vi "Bundle AOL parameters at start.vi"(6 "Case name string":string, 8 "error in (no error)":errorcluster) -> (0 "error out":errorcluster, 2 "cancelled":bool)   [LabVIEW 2020]
uses:
  Typedefs/Imaging Protocols enum.ctl
  Typedefs/AOL modes.ctl
  Global Variables/gl_UI Ctrl Refs.vi
  Global Variables/General Globals.vi
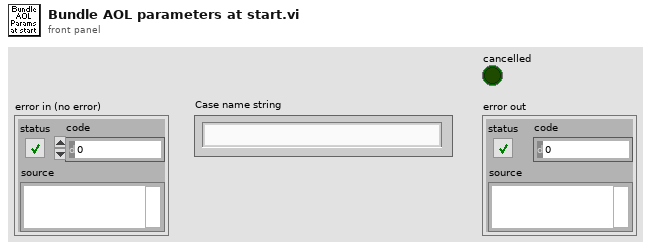
[diagram p1: front panel]
types:
  T1 = typedef "Imaging Protocols enum.ctl" = enum16{"AOL Z-Stack", "Motor Z Stack", "Parameter Sweep", "Functional Acquisition", "Single Plane Acquisition", "Volume Acquisition", "Live Imaging", "Live Plane Imaging", "Live Volume Imaging"}
  T2 = typedef "AOL modes.ctl" = enum16{"Raster", "Structural", "Pointing", "Mini Scan", "Alignment"}
  T3 = typedef "UI ctrl refs cluster.ctl" = cluster{"Top level VI path":path, "Top level VI ref":refnum<vi>, "User menu ref":refnum<k9>, "Sub Panel control":refnum<vi>, "Imaging Param Tab":refnum<vi>, "Occurrence-Start drivers":refnum<k4>, "Occurrence-Speed logging initialised":refnum<k4>, "Occurrence-XYZ stage initialised":refnum<k4>, "Exit button":refnum<vi>, "Status ind":refnum<vi>, "Set as origin":refnum<vi>, "Speed Logging":refnum<vi>, "Time Lapse":refnum<vi>, "Live Imaging":refnum<vi>, "AOL Z Stack":refnum<vi>, "Motor Z Stack":refnum<vi>, "Funct Acq button":refnum<vi>, "Hard Shutter":refnum<vi>, "Virtual Shutter":refnum<vi>, "Laser Power":refnum<vi>, "AOL Mode":refnum<vi>, "Frame Size":refnum<vi>, "Field of View":refnum<vi>, "Dwell Time":refnum<vi>, "Zoom":refnum<vi>, "AOL Z":refnum<vi>, "Objective":refnum<vi>, "Axis":refnum<vi>, "Paths & Names":refnum<vi>, "Experiment folder path (ind.)":refnum<vi>, "Last State (Ind.)":refnum<vi>, "Averages":refnum<vi>, "Angle (degrees)":refnum<vi>, "X centre":refnum<vi>, "Y centre":refnum<vi>, "Plane Mode":refnum<vi>, "# Planes":refnum<vi>, "Z Start":refnum<vi>, "Z Stop":refnum<vi>, "Z Step":refnum<vi>, "PMT 1":refnum<vi>, "PMT 2":refnum<vi>, "Stage XYZ Position":refnum<vi>, "Pockels@Z Start":refnum<vi>, "Pockels@Z Stop":refnum<vi>, "Obtain Z Start":refnum<vi>, "Obtain Z Stop":refnum<vi>, "Live stim.trig.period":refnum<vi>, "Live stim.trig.enable":refnum<vi>, "Movement Correction":refnum<vi>, "Load Reference Image":refnum<vi>, "XY Stage Move":refnum<vi>, "MovCor Cluster":refnum<vi>, "RefDAQParam":refnum<vi>, "Funct. Acq. Pockels Modulation":refnum<vi>, "Ref Laser Power":refnum<vi>, "Enable Video Recording":refnum<vi>, "Video Record-Live Imaging":refnum<vi>, "Video Record-Funct acq":refnum<vi>, "Reference Source":refnum<vi>, "AOL Z-stack Chirps Ready (ind)":refnum<vi>, "Target time between mov.cor. ref triggers (ms)":refnum<vi>, "Funct. Acq. Ref frame save":refnum<vi>, "Tracking button":refnum<vi>, "Show ref plots window":refnum<vi>, "Center freq ind (nm)":refnum<vi>, "Pickup mode (ind)":refnum<vi>, "Logging queue (ind)":refnum<vi>, "Back aperture power (ind.)":refnum<vi>, "Power after objective (ind.)":refnum<vi>, "Switch user":refnum<vi>, "Ls1 Conn. Status":refnum<vi>, "Ls1Tuning Status":refnum<vi>, "Ls1 Faults":refnum<vi>, "Ls1 Connection":refnum<vi>, "Ls1 Mode":refnum<vi>, "Ls1 POWER [mW]":refnum<vi>, "Ls1Shutter":refnum<vi>, "Ls1 Wavelength":refnum<vi>, "Ls1 Note":refnum<vi>, "Ls1 Confirm Wav":refnum<vi>, "Ls1 PreChrp Prism1":refnum<vi>, "Ls1 PreChrp Prism2":refnum<vi>, "Ls1 wav top Ind":refnum<vi>, "Ls1 power top Ind":refnum<vi>, "Ls1 Pump peak Hold":refnum<vi>, "Ls1 Status Ind":refnum<vi>, "Ls1 wav cancel":refnum<vi>, "Experiment Type":refnum<vi>, "Biology Information":refnum<vi>, "Camera recording status":refnum<vi>, "Optimise Obj. Pos.":refnum<vi>}
  T4 = typedef "AOL_Globals.ctl" = cluster{"Imaging Protocol":T1, "Number of POI":u16, "Number of Miniscans":u16, "Number of Trials":u16, "Number of Cycles ":u64, "# Averaged Frames":u16, "Laser power (%)":u8, "Pockels (V)":dbl, "Acquisition Length (sec)":dbl, "Fill time (us)":dbl, "POI Dwell time (us)":dbl, "Miniscan Dwell time per pixel (us)":dbl, "PMT 1":dbl, "PMT 2":dbl, "Back Apperture (mA)":dbl, "Frame Size":T5, "Center Frequency":dbl, "Field of View (um)":dbl, "Field of View (norm)":dbl, "DwellTime (us)":dbl, "Ref Dwell Time (us)":dbl, "Wavelength (nm)":dbl, "Zoom":dbl, "AOL Z":dbl, "AOL Mode":T2, "GridXY":dbl, "GridZ":dbl, "TriggerPeriod (sec)":dbl, "Number of Pixels in Miniscan":u16, "Experiment folder path":path, "X centre":dbl, "Y centre":dbl, "Angle (degrees)":dbl, "Angle Xs (degrees)":dbl, "Angle Ys (degrees)":dbl, "Plane Mode":T6, "Threshold":u16[], "Regenerate Chirps":bool, "Rectangle ROI length (pixels)":u16, "Rectangle ROI height (pixels)":u16, "AOD fill":u16, "StartupDelay":i32, "Samples Wait after Trigger":u16, "Slip Cycle":u32, "Add Cycle":bool, "Functional Mode":T7, "Z Start":dbl, "Z Stop":dbl, "# Planes":i32, "Total Pixels":i32, "Variable Miniscan Pixels":u16[], "Use Variable Length":bool, "Use Variable Resolution":bool, "Laser power (%) at Z Start":u8, "Laser power (%) at Z Stop":u8, "Ref Z Step":i8}
  T5 = typedef "Frame Size.ctl" = u16
  T6 = typedef "Plane Mode.ctl" = u16
  T7 = typedef "Functional Mode.ctl" = enum16{"Point", "Line", "Patch", "Plane", "Volume"}
  T8 = typedef "Laser control knob.ctl" = u16
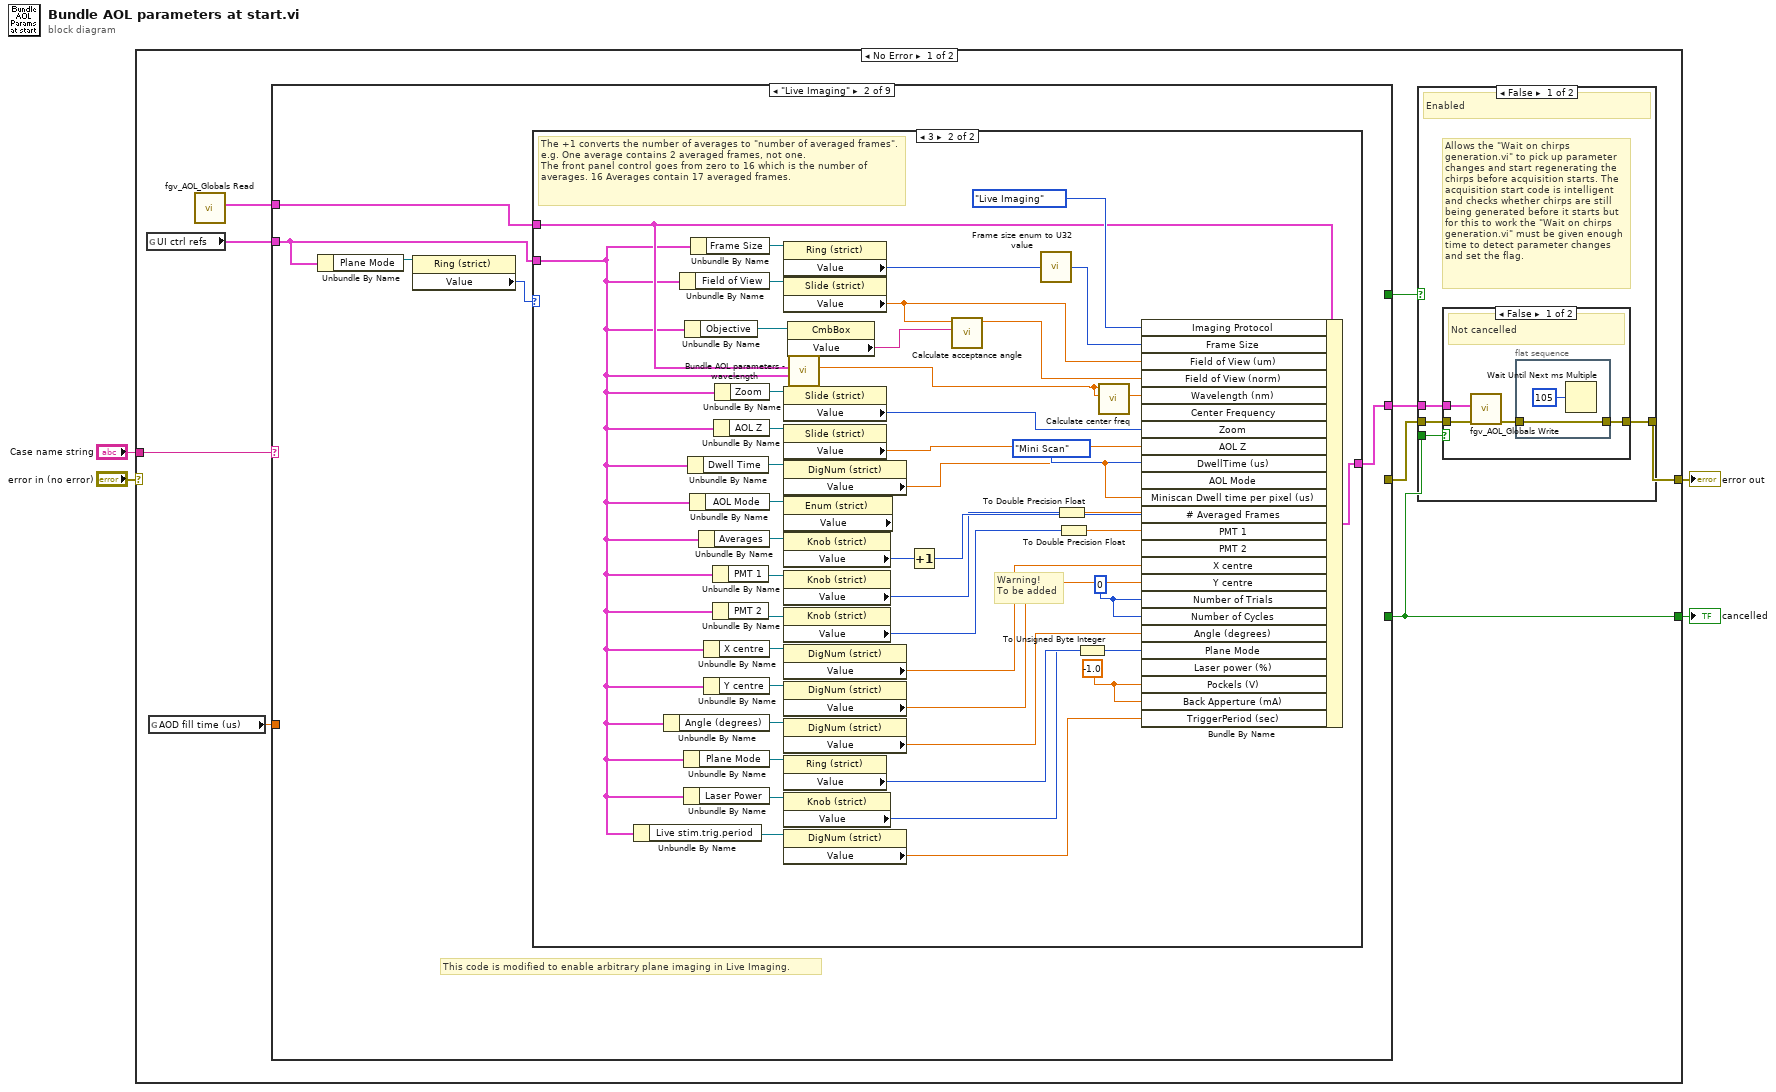
[diagram p0: block diagram]
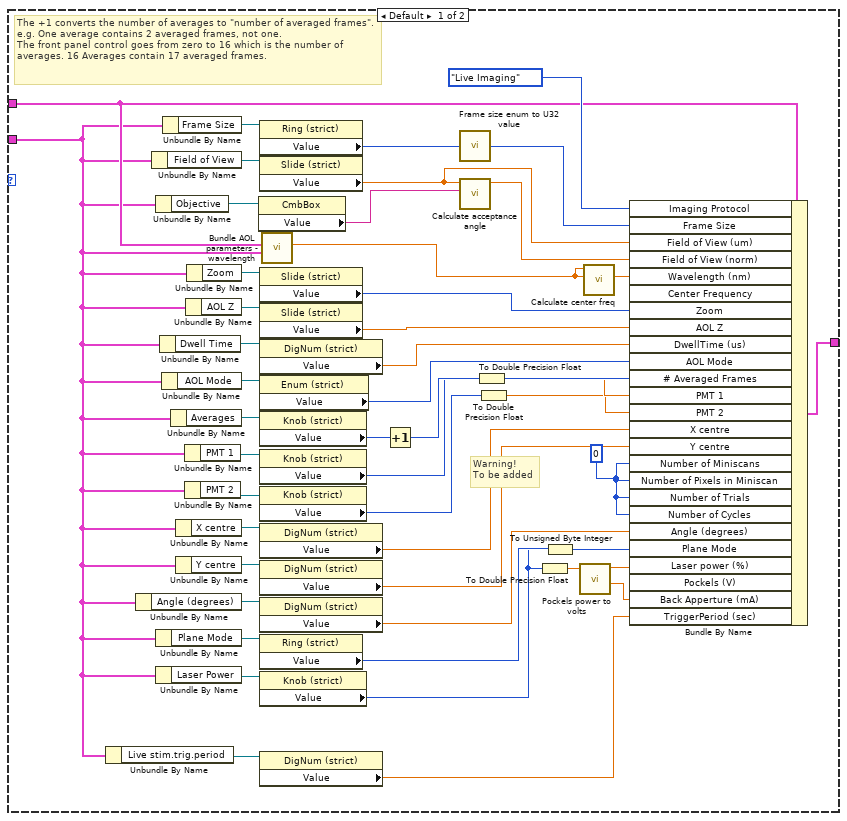
[diagram p5: hidden frame]
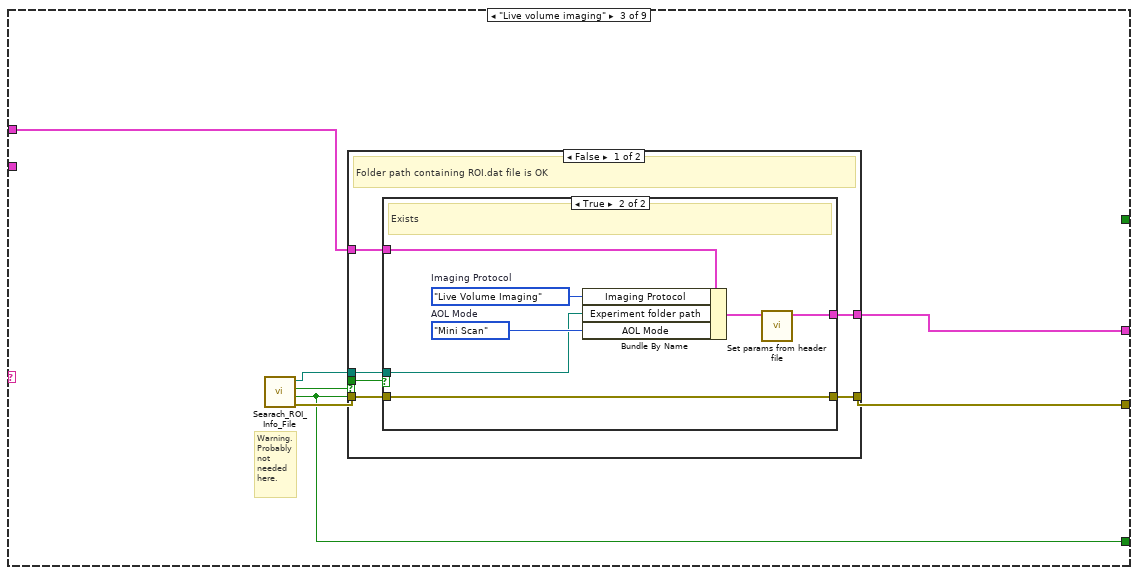
[diagram p6: hidden frame]
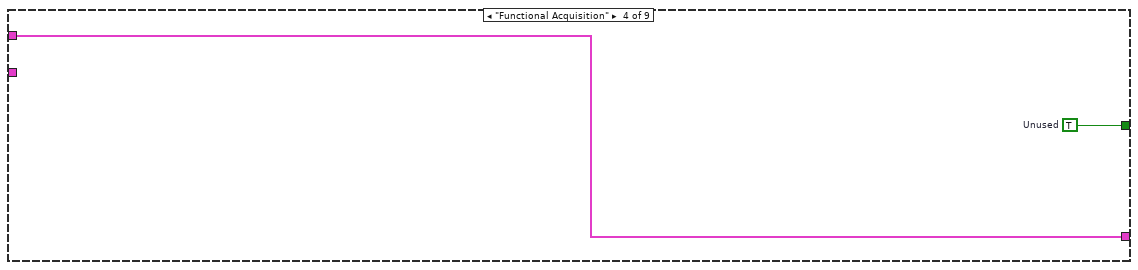
[diagram p9: hidden frame]
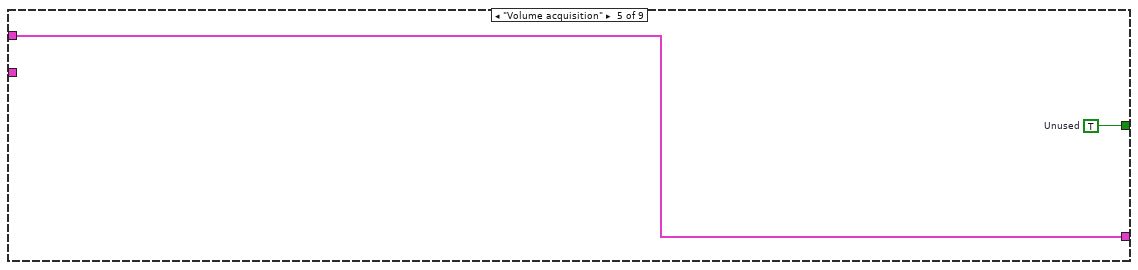
[diagram p10: hidden frame]
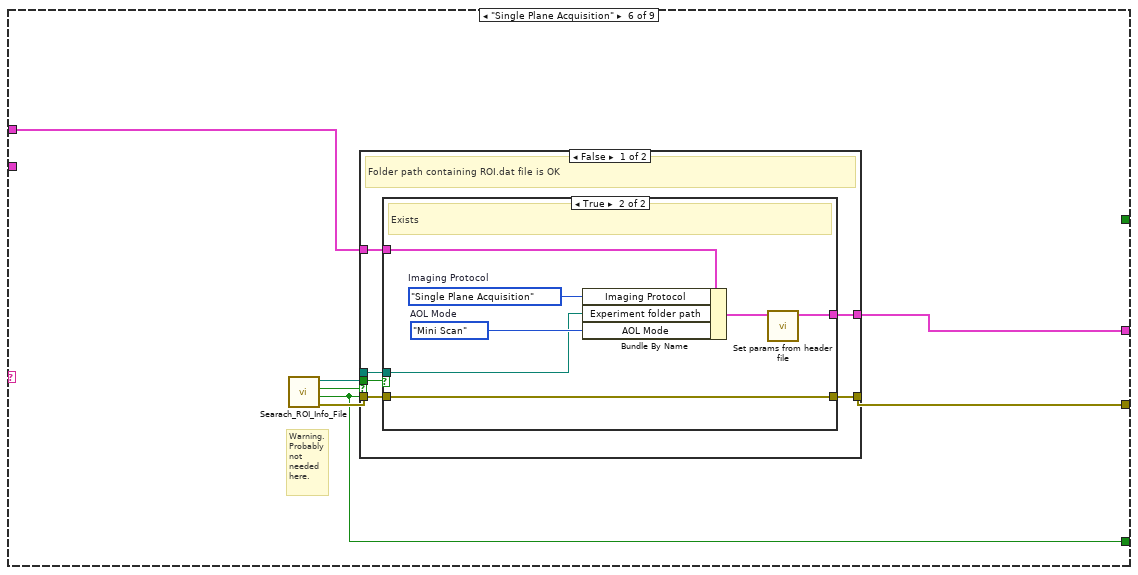
[diagram p11: hidden frame]
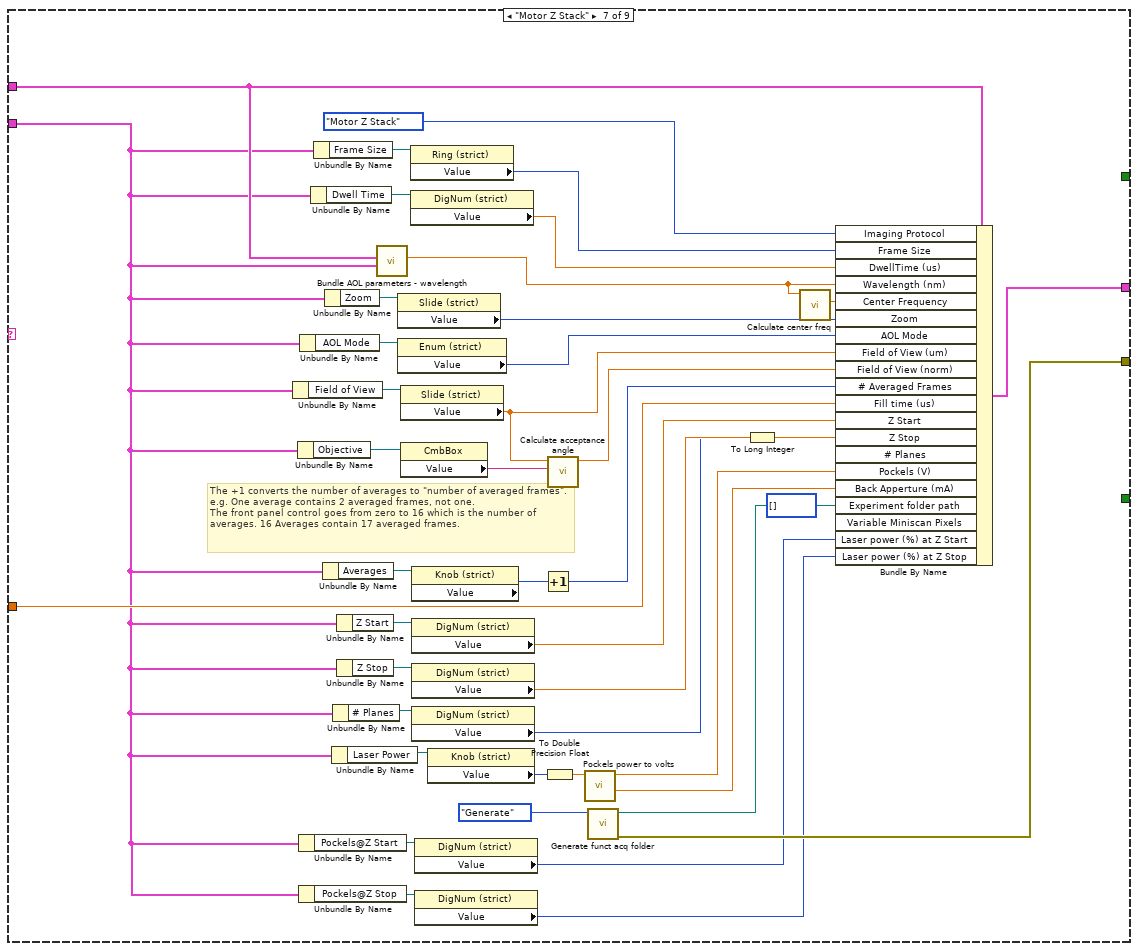
[diagram p14: hidden frame]
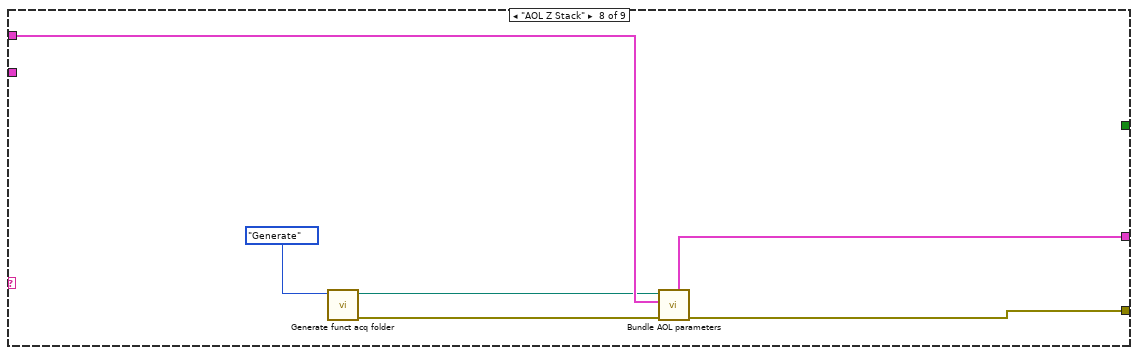
[diagram p15: hidden frame]
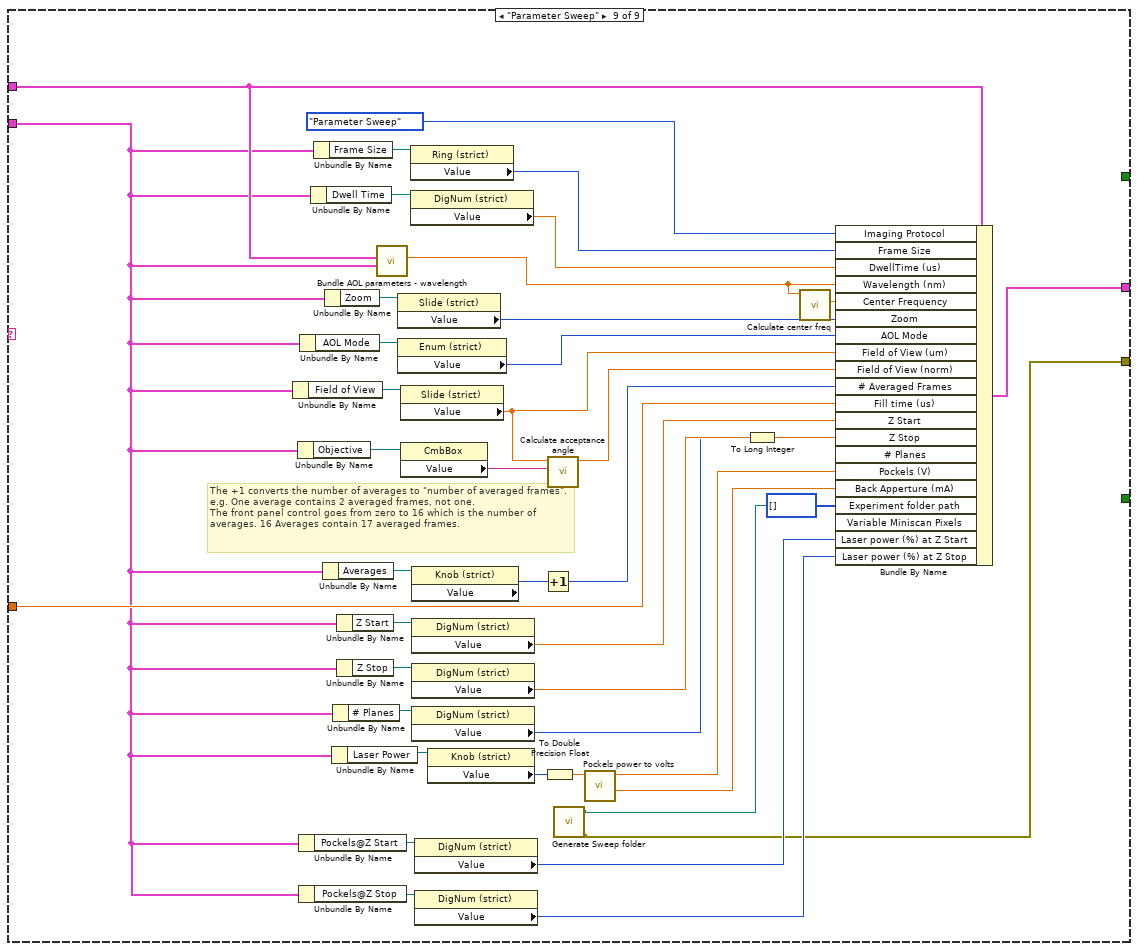
[diagram p16: hidden frame]
diagram:
  n1 = case shown="No Error" "error in (no error)" {
    selector: "error in (no error)" -> [_ w267]
    tunnel: [w13 w267] -> w1
    tunnel: "Case name string" -> [w10 _]
    tunnel: [w6 _] -> w2
    frame No Error {
      n2 = global read "gl_UI Ctrl Refs.vi" "UI ctrl refs"() -> (w9:T3)
      n3 = global read "General Globals.vi" "AOD fill time (us)"() -> (w8:dbl)
      n4 = call "fgv_AOL_Globals Read.vi"() -> ("AOL_Globals"=w11:T4)  [unwired: 9 in, 2 out]
      n5 = case shown="\"Live Imaging\"" w10 {
        tunnel: [w25 w29 w127 w149 w152 w155 w203 w222 w251] -> w12
        tunnel: w11 -> [w25 w30 w128 w149 w152 w156 w194 w223 w243]
        tunnel: w9 -> [_ w28 _ _ _ _ w180 _ w230]
        tunnel: w8 -> [_ _ _ _ _ _ w200 _ w249]
        tunnel: [_ _ w126 _ _ w154 w202 w221 w227] -> w7
        tunnel: [_ _ w125 _ _ w153 _ _ _] -> w6
        tunnel: [_ _ _ w150 w151 _ _ _ _] -> w5
        frame Default {
        }
        frame "Live Imaging" {
          # "This code is modified to enable arbitrary plane imaging in Live Imaging."
          n6 = Unbundle By Name(w28) -> ("Plane Mode"=w27:refnum<vi>)
          n7 = property on="Property Node" class="Ring (strict)"(reference=w27) -> ("Value"=w26:T6)  [unwired: 1 in, 2 out]
          n8 = case shown="3" w26 {
            tunnel: w30 -> [w41 w83]
            tunnel: [w57 w104] -> w29
            tunnel: w28 -> [w37 w79]
            frame Default {
              w78 = u16 0 ("Number of Miniscans")
              # "Warning!\nTo be added"
              # "The +1 converts the number of averages to \"number of averaged frames\". e.g. One average contains 2 averaged frames, not one.\nThe front panel control goes from zero to 16 which is the number of averages. 16 Averages contain 17 averaged frames."
              n9 = Unbundle By Name(w37) -> ("Live stim.trig.period"=w45:refnum<vi>)
              n10 = Unbundle By Name(w37) -> ("Angle (degrees)"=w61:refnum<vi>)
              n11 = Unbundle By Name(w37) -> ("Field of View"=w67:refnum<vi>)
              n12 = Unbundle By Name(w37) -> ("Objective"=w39:refnum<vi>)
              n13 = Unbundle By Name(w37) -> ("Plane Mode"=w58:refnum<vi>)
              n14 = Unbundle By Name(w37) -> ("Laser Power"=w53:refnum<vi>)
              n15 = Unbundle By Name(w37) -> ("Dwell Time"=w64:refnum<vi>)
              n16 = Unbundle By Name(w37) -> ("AOL Mode"=w63:refnum<vi>)
              n17 = Unbundle By Name(w37) -> ("Frame Size"=w68:refnum<vi>)
              n18 = Unbundle By Name(w37) -> ("Averages"=w62:refnum<vi>)
              n19 = Unbundle By Name(w37) -> ("X centre"=w60:refnum<vi>)
              n20 = Unbundle By Name(w37) -> ("Y centre"=w59:refnum<vi>)
              n21 = Unbundle By Name(w37) -> ("PMT 1"=w51:refnum<vi>)
              n22 = Unbundle By Name(w37) -> ("PMT 2"=w50:refnum<vi>)
              n23 = Unbundle By Name(w37) -> ("AOL Z"=w65:refnum<vi>)
              n24 = Unbundle By Name(w37) -> ("Zoom"=w66:refnum<vi>)
              n25 = property on="Property Node" class="CmbBox"(reference=w39) -> ("Value"=w38:string)  [unwired: 1 in, 2 out]
              n26 = property on="Property Node" class="Ring (strict)"(reference=w68) -> ("Value"=w55:T5)  [unwired: 1 in, 2 out]
              n27 = property on="Property Node" class="Slide (strict)"(reference=w67) -> ("Value"=w31:sgl)  [unwired: 1 in, 2 out]
              n28 = property on="Property Node" class="Slide (strict)"(reference=w66) -> ("Value"=w73:i8)  [unwired: 1 in, 2 out]
              n29 = property on="Property Node" class="Slide (strict)"(reference=w65) -> ("Value"=w70:sgl)  [unwired: 1 in, 2 out]
              n30 = property on="Property Node" class="DigNum (strict)"(reference=w64) -> ("Value"=w71:dbl)  [unwired: 1 in, 2 out]
              n31 = property on="Property Node" class="Enum (strict)"(reference=w63) -> ("Value"=w77:T2)  [unwired: 1 in, 2 out]
              n32 = property on="Property Node" class="Knob (strict)"(reference=w62) -> ("Value"=w72:u16)  [unwired: 1 in, 2 out]
              n33 = property on="Property Node" class="Knob (strict)"(reference=w51) -> ("Value"=w49:T8)  [unwired: 1 in, 2 out]
              n34 = property on="Property Node" class="Knob (strict)"(reference=w50) -> ("Value"=w48:T8)  [unwired: 1 in, 2 out]
              n35 = property on="Property Node" class="DigNum (strict)"(reference=w60) -> ("Value"=w74:dbl)  [unwired: 1 in, 2 out]
              n36 = property on="Property Node" class="DigNum (strict)"(reference=w59) -> ("Value"=w75:dbl)  [unwired: 1 in, 2 out]
              n37 = property on="Property Node" class="DigNum (strict)"(reference=w61) -> ("Value"=w69:dbl)  [unwired: 1 in, 2 out]
              n38 = property on="Property Node" class="Ring (strict)"(reference=w58) -> ("Value"=w43:T6)  [unwired: 1 in, 2 out]
              n39 = property on="Property Node" class="Knob (strict)"(reference=w53) -> ("Value"=w33:T8)  [unwired: 1 in, 2 out]
              n40 = property on="Property Node" class="DigNum (strict)"(reference=w45) -> ("Value"=w44:dbl)  [unwired: 1 in, 2 out]
              n41 = call "Bundle AOL parameters - wavelength.vi"("UI ctrl refs"=w37, "AOL_Globals in"=w41) -> ("Wavelength"=w40:dbl)  [unwired: 9 in]
              n42 = Increment(x=w72) -> (x+1=w56:u16)
              n43 = call "Frame size enum to U32 value.vi"("Value"=w55) -> ("Frame Size U32"=w54:u32)
              n44 = call "Calculate acceptance angle.vi"("Objective"=w38, "FOV (true)"=w31) -> ("Acceptance Angle (mrad)"=w36:dbl)  [unwired: 8 in, 1 out]
              n45 = To Double Precision Float(number=w49) -> (double precision float=w47:dbl)
              n46 = To Double Precision Float(number=w48) -> (double precision float=w46:dbl)
              n47 = To Double Precision Float(number=w33) -> (double precision float=w32:dbl)
              n48 = To Unsigned Byte Integer(number=w33) -> (unsigned 8bit integer=w52:u8)
              n49 = call "Pockels power to volts.vi"("Pockels power (%)"=w32) -> ("Back-aperture power (mW)"=w34:dbl, "Pockels control voltage (V)"=w35:dbl)  [unwired: 8 in, 1 out]
              n50 = call "Calculate center freq.vi"("UI Wavelength"=w40) -> ("Centre frequency (MHz)"=w42:dbl)  [unwired: 9 in, 1 out]
              n51 = Bundle By Name(cluster=w41, "Imaging Protocol"=Imaging_Protocols_enum."Live Imaging" ("Imaging Mode"), "Frame Size"=w54, "Field of View (um)"=w31, "Field of View (norm)"=w36, "Wavelength (nm)"=w40, "Center Frequency"=w42, "Zoom"=w73, "AOL Z"=w70, "DwellTime (us)"=w71, "AOL Mode"=w77, "# Averaged Frames"=w56, "PMT 1"=w47, "PMT 2"=w46, "X centre"=w74, "Y centre"=w75, "Number of Miniscans"=w78, "Number of Pixels in Miniscan"=w78, "Number of Trials"=w78, "Number of Cycles"=w78, "Angle (degrees)"=w69, "Plane Mode"=w43, "Laser power (%)"=w52, "Pockels (V)"=w35, "Back Apperture (mA)"=w34, "TriggerPeriod (sec)"=w44) -> (w57:T4)
            }
            frame 3 {
              w91 = -1.0 ("Pockels")
              w124 = u16 0 ("Number of Miniscans")
              # "Warning!\nTo be added"
              # "The +1 converts the number of averages to \"number of averaged frames\". e.g. One average contains 2 averaged frames, not one.\nThe front panel control goes from zero to 16 which is the number of averages. 16 Averages contain 17 averaged frames."
              n52 = Unbundle By Name(w79) -> ("Live stim.trig.period"=w89:refnum<vi>)
              n53 = Unbundle By Name(w79) -> ("Angle (degrees)"=w108:refnum<vi>)
              n54 = Unbundle By Name(w79) -> ("Field of View"=w114:refnum<vi>)
              n55 = Unbundle By Name(w79) -> ("Plane Mode"=w105:refnum<vi>)
              n56 = Unbundle By Name(w79) -> ("Laser Power"=w100:refnum<vi>)
              n57 = Unbundle By Name(w79) -> ("Objective"=w84:refnum<vi>)
              n58 = Unbundle By Name(w79) -> ("Dwell Time"=w111:refnum<vi>)
              n59 = Unbundle By Name(w79) -> ("AOL Mode"=w110:refnum<vi>)
              n60 = Unbundle By Name(w79) -> ("Frame Size"=w115:refnum<vi>)
              n61 = Unbundle By Name(w79) -> ("Averages"=w109:refnum<vi>)
              n62 = Unbundle By Name(w79) -> ("X centre"=w107:refnum<vi>)
              n63 = Unbundle By Name(w79) -> ("Y centre"=w106:refnum<vi>)
              n64 = Unbundle By Name(w79) -> ("PMT 1"=w97:refnum<vi>)
              n65 = Unbundle By Name(w79) -> ("PMT 2"=w96:refnum<vi>)
              n66 = Unbundle By Name(w79) -> ("AOL Z"=w112:refnum<vi>)
              n67 = Unbundle By Name(w79) -> ("Zoom"=w113:refnum<vi>)
              n68 = property on="Property Node" class="Ring (strict)"(reference=w115) -> ("Value"=w102:T5)  [unwired: 1 in, 2 out]
              n69 = property on="Property Node" class="Slide (strict)"(reference=w114) -> ("Value"=w82:sgl)  [unwired: 1 in, 2 out]
              n70 = property on="Property Node" class="Slide (strict)"(reference=w113) -> ("Value"=w120:i8)  [unwired: 1 in, 2 out]
              n71 = property on="Property Node" class="Slide (strict)"(reference=w112) -> ("Value"=w118:sgl)  [unwired: 1 in, 2 out]
              n72 = property on="Property Node" class="DigNum (strict)"(reference=w111) -> ("Value"=w87:dbl)  [unwired: 1 in, 2 out]
              n73 = property on="Property Node" class="Enum (strict)" props=["Value"](reference=w110) -> ()  [unwired: 1 in, 3 out]
              n74 = property on="Property Node" class="Knob (strict)"(reference=w109) -> ("Value"=w119:u16)  [unwired: 1 in, 2 out]
              n75 = property on="Property Node" class="Knob (strict)"(reference=w97) -> ("Value"=w95:T8)  [unwired: 1 in, 2 out]
              n76 = property on="Property Node" class="Knob (strict)"(reference=w96) -> ("Value"=w94:T8)  [unwired: 1 in, 2 out]
              n77 = property on="Property Node" class="DigNum (strict)"(reference=w107) -> ("Value"=w121:dbl)  [unwired: 1 in, 2 out]
              n78 = property on="Property Node" class="DigNum (strict)"(reference=w106) -> ("Value"=w122:dbl)  [unwired: 1 in, 2 out]
              n79 = property on="Property Node" class="DigNum (strict)"(reference=w108) -> ("Value"=w117:dbl)  [unwired: 1 in, 2 out]
              n80 = property on="Property Node" class="Ring (strict)"(reference=w105) -> ("Value"=w116:T6)  [unwired: 1 in, 2 out]
              n81 = property on="Property Node" class="Knob (strict)"(reference=w100) -> ("Value"=w99:T8)  [unwired: 1 in, 2 out]
              n82 = property on="Property Node" class="DigNum (strict)"(reference=w89) -> ("Value"=w88:dbl)  [unwired: 1 in, 2 out]
              n83 = property on="Property Node" class="CmbBox"(reference=w84) -> ("Value"=w81:string)  [unwired: 1 in, 2 out]
              n84 = call "Bundle AOL parameters - wavelength.vi"("UI ctrl refs"=w79, "AOL_Globals in"=w83) -> ("Wavelength"=w85:dbl)  [unwired: 9 in]
              n85 = Increment(x=w119) -> (x+1=w103:u16)
              n86 = call "Calculate acceptance angle.vi"("Objective"=w81, "FOV (true)"=w82) -> ("Acceptance Angle (mrad)"=w80:dbl)  [unwired: 8 in, 1 out]
              n87 = call "Frame size enum to U32 value.vi"("Value"=w102) -> ("Frame Size U32"=w101:u32)
              n88 = To Double Precision Float(number=w95) -> (double precision float=w93:dbl)
              n89 = To Double Precision Float(number=w94) -> (double precision float=w92:dbl)
              n90 = To Unsigned Byte Integer(number=w99) -> (unsigned 8bit integer=w98:u8)
              n91 = call "Calculate center freq.vi"("UI Wavelength"=w85) -> ("Centre frequency (MHz)"=w86:dbl)  [unwired: 9 in, 1 out]
              n92 = Bundle By Name(cluster=w83, "Imaging Protocol"=Imaging_Protocols_enum."Live Imaging" ("Imaging Mode"), "Frame Size"=w101, "Field of View (um)"=w82, "Field of View (norm)"=w80, "Wavelength (nm)"=w85, "Center Frequency"=w86, "Zoom"=w120, "AOL Z"=w118, "DwellTime (us)"=w87, "AOL Mode"=AOL_modes."Mini Scan", "Miniscan Dwell time per pixel (us)"=w87, "# Averaged Frames"=w103, "PMT 1"=w93, "PMT 2"=w92, "X centre"=w121, "Y centre"=w122, "Number of Trials"=w124, "Number of Cycles"=w124, "Angle (degrees)"=w117, "Plane Mode"=w116, "Laser power (%)"=w98, "Pockels (V)"=w91, "Back Apperture (mA)"=w91, "TriggerPeriod (sec)"=w88) -> (w104:T4)
            }
          }
        }
        frame "Live volume imaging" {
          # "Warning.\nProbably not needed here."
          n93 = call "Searach_ROI_Info_File.vi"() -> ("error out"=w130:errorcluster, "cancelled"=w125:bool, "exists"=w129:bool, "Experiment folder"=w131:path)  [unwired: 8 in]
          n94 = case shown="False" w125 {
            tunnel: w131 -> [w137 _]
            tunnel: w130 -> [w136 w147]
            tunnel: w129 -> [w135 _]
            tunnel: w128 -> [w134 w148]
            tunnel: [w133 w148] -> w127
            tunnel: [w132 w147] -> w126
            frame False {
              # "Folder path containing ROI.dat file is OK"
              n95 = case shown="True" w135 {
                tunnel: w137 -> [_ w144]
                tunnel: w136 -> [w139 w141]
                tunnel: w134 -> [w138 w143]
                tunnel: [w138 w140] -> w133
                tunnel: [w139 w141] -> w132
                frame False {
                  # "Deos not exist"
                }
                frame True {
                  w145 = AOL_modes."Mini Scan"  # AOL Mode
                  w146 = Imaging_Protocols_enum."Live Volume Imaging"  # Imaging Protocol
                  # "Exists"
                  n96 = Bundle By Name(cluster=w143, "Imaging Protocol"=w146, "Experiment folder path"=w144, "AOL Mode"=w145) -> (w142:T4)
                  n97 = call "Set params from header file.vi"("AOL_Globals in"=w142) -> ("AOL_Globals out"=w140:T4)  [unwired: 10 in]
                }
              }
            }
            frame True {
              # "Cancelled"
            }
          }
        }
        frame "Functional Acquisition" {
          w150 = TRUE  # Unused
        }
        frame "Volume acquisition" {
          w151 = TRUE  # Unused
        }
        frame "Single Plane Acquisition" {
          # "Warning.\nProbably not needed here."
          n98 = call "Searach_ROI_Info_File.vi"() -> ("error out"=w158:errorcluster, "cancelled"=w153:bool, "exists"=w157:bool, "Experiment folder"=w159:path)  [unwired: 8 in]
          n99 = case shown="False" w153 {
            tunnel: w159 -> [w165 _]
            tunnel: w158 -> [w164 w175]
            tunnel: w157 -> [w163 _]
            tunnel: w156 -> [w162 w176]
            tunnel: [w161 w176] -> w155
            tunnel: [w160 w175] -> w154
            frame False {
              # "Folder path containing ROI.dat file is OK"
              n100 = case shown="True" w163 {
                tunnel: w165 -> [_ w172]
                tunnel: w164 -> [w167 w170]
                tunnel: w162 -> [w166 w171]
                tunnel: [w166 w168] -> w161
                tunnel: [w167 w170] -> w160
                frame False {
                  # "Deos not exist"
                }
                frame True {
                  w173 = AOL_modes."Mini Scan"  # AOL Mode
                  w174 = Imaging_Protocols_enum."Single Plane Acquisition"  # Imaging Protocol
                  # "Exists"
                  n101 = Bundle By Name(cluster=w171, "Imaging Protocol"=w174, "Experiment folder path"=w172, "AOL Mode"=w173) -> (w169:T4)
                  n102 = call "Set params from header file.vi"("AOL_Globals in"=w169) -> ("AOL_Globals out"=w168:T4)  [unwired: 10 in]
                }
              }
            }
            frame True {
              # "Cancelled"
            }
          }
        }
        frame "Motor Z Stack" {
          # "The +1 converts the number of averages to \"number of averaged frames\". e.g. One average contains 2 averaged frames, not one.\nThe front panel control goes from zero to 16 which is the number of averages. 16 Averages contain 17 averaged frames."
          n103 = Unbundle By Name(w180) -> ("Field of View"=w212:refnum<vi>)
          n104 = Unbundle By Name(w180) -> ("Objective"=w192:refnum<vi>)
          n105 = Unbundle By Name(w180) -> ("Pockels@Z Start"=w182:refnum<vi>)
          n106 = Unbundle By Name(w180) -> ("Pockels@Z Stop"=w181:refnum<vi>)
          n107 = Unbundle By Name(w180) -> ("AOL Mode"=w213:refnum<vi>)
          n108 = Unbundle By Name(w180) -> ("Dwell Time"=w215:refnum<vi>)
          n109 = Unbundle By Name(w180) -> ("Frame Size"=w217:refnum<vi>)
          n110 = Unbundle By Name(w180) -> ("Averages"=w211:refnum<vi>)
          n111 = Unbundle By Name(w180) -> ("Zoom"=w214:refnum<vi>)
          n112 = Unbundle By Name(w180) -> ("Laser Power"=w188:refnum<vi>)
          n113 = Unbundle By Name(w180) -> ("# Planes"=w207:refnum<vi>)
          n114 = Unbundle By Name(w180) -> ("Z Start"=w205:refnum<vi>)
          n115 = Unbundle By Name(w180) -> ("Z Stop"=w206:refnum<vi>)
          n116 = call "Bundle AOL parameters - wavelength.vi"("UI ctrl refs"=w180, "AOL_Globals in"=w194) -> ("Wavelength"=w193:dbl)  [unwired: 9 in]
          n117 = property class="Slide (strict)"(reference=w214) -> ("Value"=w204:i8)  [unwired: 1 in, 2 out]
          n118 = property class="Enum (strict)"(reference=w213) -> ("Value"=w209:T2)  [unwired: 1 in, 2 out]
          n119 = property class="Slide (strict)"(reference=w212) -> ("Value"=w177:sgl)  [unwired: 1 in, 2 out]
          n120 = property on="Property Node" class="CmbBox"(reference=w192) -> ("Value"=w191:string)  [unwired: 1 in, 2 out]
          n121 = property class="Ring (strict)"(reference=w217) -> ("Value"=w216:u16)  [unwired: 1 in, 2 out]
          n122 = property class="DigNum (strict)"(reference=w215) -> ("Value"=w210:dbl)  [unwired: 1 in, 2 out]
          n123 = property class="Knob (strict)"(reference=w211) -> ("Value"=w208:u16)  [unwired: 1 in, 2 out]
          n124 = property class="DigNum (strict)"(reference=w205) -> ("Value"=w198:dbl)  [unwired: 1 in, 2 out]
          n125 = property class="DigNum (strict)"(reference=w206) -> ("Value"=w197:dbl)  [unwired: 1 in, 2 out]
          n126 = property class="DigNum (strict)"(reference=w207) -> ("Value"=w195:u16)  [unwired: 1 in, 2 out]
          n127 = property on="Property Node" class="DigNum (strict)"(reference=w182) -> ("Value"=w179:u16)  [unwired: 1 in, 2 out]
          n128 = property on="Property Node" class="DigNum (strict)"(reference=w181) -> ("Value"=w178:u16)  [unwired: 1 in, 2 out]
          n129 = property class="Knob (strict)"(reference=w188) -> ("Value"=w186:T8)  [unwired: 1 in, 2 out]
          n130 = Increment(x=w208) -> (x+1=w201:u16)
          n131 = To Double Precision Float(number=w186) -> (double precision float=w187:dbl)
          n132 = call "Calculate acceptance angle.vi"("Objective"=w191, "FOV (true)"=w177) -> ("Acceptance Angle (mrad)"=w190:dbl)  [unwired: 8 in, 1 out]
          n133 = call "Pockels power to volts.vi"("Pockels power (%)"=w187) -> ("Back-aperture power (mW)"=w184:dbl, "Pockels control voltage (V)"=w185:dbl)  [unwired: 8 in, 1 out]
          n134 = call "Generate funct acq folder.vi"("Function"=enum16{"Generate", "Obtain"}."Generate") -> ("error out"=w202:errorcluster, "Funct acq experiment folder path"=w189:path)  [unwired: 9 in]
          n135 = To Long Integer(number=w195) -> (32bit integer=w196:i32)
          n136 = call "Calculate center freq.vi"("UI Wavelength"=w193) -> ("Centre frequency (MHz)"=w199:dbl)  [unwired: 9 in, 1 out]
          n137 = Bundle By Name(cluster=w194, "Imaging Protocol"=Imaging_Protocols_enum."Motor Z Stack" ("Imaging Mode"), "Frame Size"=w216, "DwellTime (us)"=w210, "Wavelength (nm)"=w193, "Center Frequency"=w199, "Zoom"=w204, "AOL Mode"=w209, "Field of View (um)"=w177, "Field of View (norm)"=w190, "# Averaged Frames"=w201, "Fill time (us)"=w200, "Z Start"=w198, "Z Stop"=w197, "# Planes"=w196, "Pockels (V)"=w185, "Back Apperture (mA)"=w184, "Experiment folder path"=w189, "Variable Miniscan Pixels"=u16[] [], "Laser power (%) at Z Start"=w179, "Laser power (%) at Z Stop"=w178) -> (w203:T4)
        }
        frame "AOL Z Stack" {
          n138 = call "Generate funct acq folder.vi"("Function"=enum16{"Generate", "Obtain"}."Generate") -> ("error out"=w221:errorcluster, "Funct acq experiment folder path"=w220:path)  [unwired: 9 in]
          n139 = call "Bundle AOL parameters.vi"("AOL_Globals in"=w223, "Experiment folder path"=w220) -> ("AOL_Globals out"=w222:T4)  [unwired: 9 in]
        }
        frame "Parameter Sweep" {
          # "The +1 converts the number of averages to \"number of averaged frames\". e.g. One average contains 2 averaged frames, not one.\nThe front panel control goes from zero to 16 which is the number of averages. 16 Averages contain 17 averaged frames."
          n140 = Unbundle By Name(w230) -> ("Field of View"=w260:refnum<vi>)
          n141 = Unbundle By Name(w230) -> ("Objective"=w241:refnum<vi>)
          n142 = Unbundle By Name(w230) -> ("Pockels@Z Start"=w232:refnum<vi>)
          n143 = Unbundle By Name(w230) -> ("Pockels@Z Stop"=w231:refnum<vi>)
          n144 = Unbundle By Name(w230) -> ("AOL Mode"=w261:refnum<vi>)
          n145 = Unbundle By Name(w230) -> ("Dwell Time"=w263:refnum<vi>)
          n146 = Unbundle By Name(w230) -> ("Frame Size"=w265:refnum<vi>)
          n147 = Unbundle By Name(w230) -> ("Averages"=w259:refnum<vi>)
          n148 = Unbundle By Name(w230) -> ("Zoom"=w262:refnum<vi>)
          n149 = Unbundle By Name(w230) -> ("Laser Power"=w238:refnum<vi>)
          n150 = Unbundle By Name(w230) -> ("# Planes"=w255:refnum<vi>)
          n151 = Unbundle By Name(w230) -> ("Z Start"=w253:refnum<vi>)
          n152 = Unbundle By Name(w230) -> ("Z Stop"=w254:refnum<vi>)
          n153 = call "Bundle AOL parameters - wavelength.vi"("UI ctrl refs"=w230, "AOL_Globals in"=w243) -> ("Wavelength"=w242:dbl)  [unwired: 9 in]
          n154 = property class="Slide (strict)"(reference=w262) -> ("Value"=w252:i8)  [unwired: 1 in, 2 out]
          n155 = property class="Enum (strict)"(reference=w261) -> ("Value"=w257:T2)  [unwired: 1 in, 2 out]
          n156 = property class="Slide (strict)"(reference=w260) -> ("Value"=w225:sgl)  [unwired: 1 in, 2 out]
          n157 = property on="Property Node" class="CmbBox"(reference=w241) -> ("Value"=w240:string)  [unwired: 1 in, 2 out]
          n158 = property class="Ring (strict)"(reference=w265) -> ("Value"=w264:u16)  [unwired: 1 in, 2 out]
          n159 = property class="DigNum (strict)"(reference=w263) -> ("Value"=w258:dbl)  [unwired: 1 in, 2 out]
          n160 = property class="Knob (strict)"(reference=w259) -> ("Value"=w256:u16)  [unwired: 1 in, 2 out]
          n161 = property class="DigNum (strict)"(reference=w253) -> ("Value"=w247:dbl)  [unwired: 1 in, 2 out]
          n162 = property class="DigNum (strict)"(reference=w254) -> ("Value"=w246:dbl)  [unwired: 1 in, 2 out]
          n163 = property class="DigNum (strict)"(reference=w255) -> ("Value"=w244:u16)  [unwired: 1 in, 2 out]
          n164 = property on="Property Node" class="DigNum (strict)"(reference=w232) -> ("Value"=w229:u16)  [unwired: 1 in, 2 out]
          n165 = property on="Property Node" class="DigNum (strict)"(reference=w231) -> ("Value"=w228:u16)  [unwired: 1 in, 2 out]
          n166 = property class="Knob (strict)"(reference=w238) -> ("Value"=w236:T8)  [unwired: 1 in, 2 out]
          n167 = Increment(x=w256) -> (x+1=w250:u16)
          n168 = To Double Precision Float(number=w236) -> (double precision float=w237:dbl)
          n169 = call "Calculate acceptance angle.vi"("Objective"=w240, "FOV (true)"=w225) -> ("Acceptance Angle (mrad)"=w239:dbl)  [unwired: 8 in, 1 out]
          n170 = call "Generate Sweep folder.vi"() -> ("error out"=w227:errorcluster, "Timelapse folder path"=w226:path)  [unwired: 10 in]
          n171 = call "Pockels power to volts.vi"("Pockels power (%)"=w237) -> ("Back-aperture power (mW)"=w234:dbl, "Pockels control voltage (V)"=w235:dbl)  [unwired: 8 in, 1 out]
          n172 = To Long Integer(number=w244) -> (32bit integer=w245:i32)
          n173 = call "Calculate center freq.vi"("UI Wavelength"=w242) -> ("Centre frequency (MHz)"=w248:dbl)  [unwired: 9 in, 1 out]
          n174 = Bundle By Name(cluster=w243, "Imaging Protocol"=Imaging_Protocols_enum."Parameter Sweep" ("Imaging Mode"), "Frame Size"=w264, "DwellTime (us)"=w258, "Wavelength (nm)"=w242, "Center Frequency"=w248, "Zoom"=w252, "AOL Mode"=w257, "Field of View (um)"=w225, "Field of View (norm)"=w239, "# Averaged Frames"=w250, "Fill time (us)"=w249, "Z Start"=w247, "Z Stop"=w246, "# Planes"=w245, "Pockels (V)"=w235, "Back Apperture (mA)"=w234, "Experiment folder path"=w226, "Variable Miniscan Pixels"=u16[] [], "Laser power (%) at Z Start"=w229, "Laser power (%) at Z Stop"=w228) -> (w251:T4)
        }
      }
      n175 = case shown="False" w5 {
        tunnel: [w17 _] -> w13
        tunnel: w12 -> [w16 _]
        tunnel: w7 -> [w15 _]
        tunnel: w6 -> [w14 _]
        frame False {
          # "Allows the\t\"Wait on chirps generation.vi\" to pick up parameter changes and start regenerating the chirps before acquisition starts. The acquisition start code is intelligent and checks whether chirps are still being generated before it starts but for this to work the \"Wait on chirps generation.vi\" must be given enough time to detect parameter changes and set the flag."
          # "Enabled"
          n176 = case shown="False" w14 {
            tunnel: [w18 w24] -> w17
            tunnel: w16 -> [w21 _]
            tunnel: w15 -> [w20 w24]
            frame False {
              # "Not cancelled"
              n177 = call "fgv_AOL_Globals Write.vi"("error in (no error)"=w20, "AOL_Globals"=w21) -> ("error out"=w19:errorcluster)  [unwired: 9 in]
              n178 = flat-sequence {
                tunnel: w19 -> [w23]
                tunnel: [w23] -> w18
                frame #0 {
                  n179 = Wait Until Next ms Multiple(millisecond multiple=u32 105) -> ()  [unwired: 1 out]
                }
              }
            }
            frame True {
              # "Cancelled"
            }
          }
        }
        frame True {
          # "Unused"
        }
      }
    }
    frame Error {
    }
  }
  "error out" <- w1
  "cancelled" <- w2
